vi "CheckQueue.vi"() -> (0 "x > 0?":bool)   [LabVIEW 2019]
uses:
  GraphsQueue.vi
  Global.lvlib
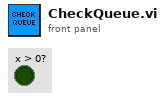
[diagram p1: front panel]
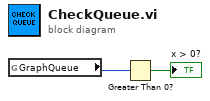
[diagram p0: block diagram]
diagram:
  n1 = global read "GraphsQueue.vi" "GraphQueue"() -> (w2:i16)
  n2 = Greater Than 0?(x=w2) -> (x > 0?=→"x > 0?":bool)
